vi "QR_code_Check.vi"(6 "Columns":string[](array[string]), 7 "format string":string, 8 "error in (no error)":errorcluster, 9 "replace %s":string, 10 "table":string, 11 "Refnum in":T1) -> (0 "error out":errorcluster, 2 "ON no barcode NOT PRESENT":bool, 3 "Refnum out":T1)   [LabVIEW 2017]
uses:
  <vilib>/addons/database/Connection.llb/Conn ObjectReference.ctl
  <vilib>/addons/database/NI_Database_API.lvlib
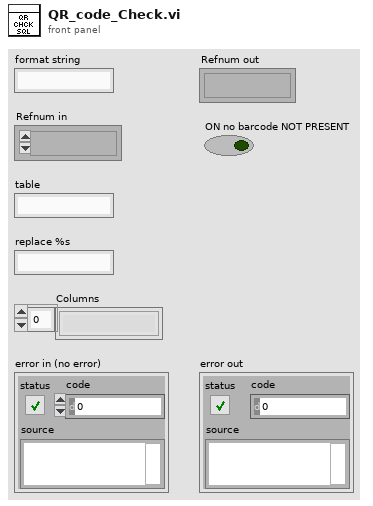
[diagram p1: front panel]
types:
  T1 = typedef "NI_Database_API.lvlib/Conn ObjectReference.ctl" = refnum<k1>
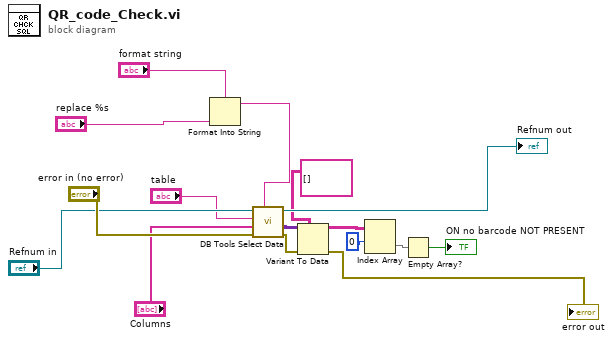
[diagram p0: block diagram]
diagram:
  n1 = Format Into String(format string="format string", "replace %s") -> (resulting string=w2:string)  [unwired: 2 in, 1 out]
  n2 = call <vilib>:"DB Tools Select Data.vi"("condition"=w2, "error in (no error)"="error in (no error)", "columns"="Columns", "table"="table", "connection reference"="Refnum in") -> ("error out"=w3:errorcluster, "data"=w5:variant[][], "connection reference out"=→"Refnum out":T1)  [unwired: 1 in]
  n3 = Variant To Data(error in=w3, type=string[][] [], Variant=w5) -> (data=w4:string[][], error out=→"error out":errorcluster)
  n4 = Index Array(array=w4, index (row)=0) -> (element=w1:string[])  [unwired: 1 in]
  n5 = Empty Array?(array=w1) -> (empty?=→"ON no barcode NOT PRESENT":bool)
